vi "Main.vi"() -> ()   [LabVIEW 2013]
uses:
  <vilib>/Utility/error.llb/DialogType.ctl
panel:
  in  "IP":string="192.168.1.4"
  in  "SetRemote":bool
  in  "Сброс ERR":bool
  in  "График":bool
  in  "Voltage 2":u8 caption="мА" max=24 step=1
  in  "SetIB":bool
  in  "Voltage":dbl caption="кВ" min=0.0 max=50.0 step=0.1 format="%.1g"
  in  "SetUB":bool
  out "Режим":bool
  out "Статус":bool
  out "Блок.":bool
  out "Uвых":dbl(graph)
  out "мА":string
  out "Выход":bool
  in  "вкл.":bool
  out "conn src":refnum<k5>
  in  "stop":bool
  out "message":string=" INSTRUCTIONS:\r\rNormal Use:  When using subVIs that incorporate the error in/error out (or error I/O) structure, place this handler where you want to inform the user of an error, typically at the end of the I/O data path, as the last action of the program.  If the error in error? is ERROR, the handler creates a message describing the error and its source.  If the type of dialog = 1 (default), the message is displayed to the user, who can only acknowedge it.  If the type = 2, the user can acknowledge the message or abort execution; aborting a program with active I/O is not recommended.  If the type = 0, no message is displayed; this is used to process the error programmatically, and the error out cluster elements are wired to individual terminals for that reason.  \r\rOther Use:\n\r\nlocal testing.  To test the error code of a subVI or function that does not have the error I/O structure, you can wire its error code and a source string to the local error code and error source inputs.  If error in error? indicates no error and error code is not equal to 0, the local code and source are substituted for the error in values, and error? is set TRUE (ERROR)."
  out "кВ":string
  # "SPELLMAN 50 кВ 24 мА"
  # "Установки"
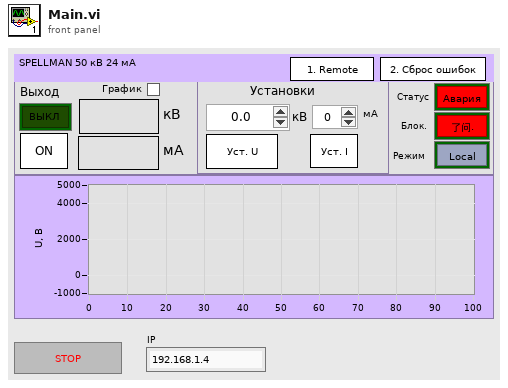
[diagram p1: front panel]
types:
  T1 = typedef "DialogType.ctl" = u16
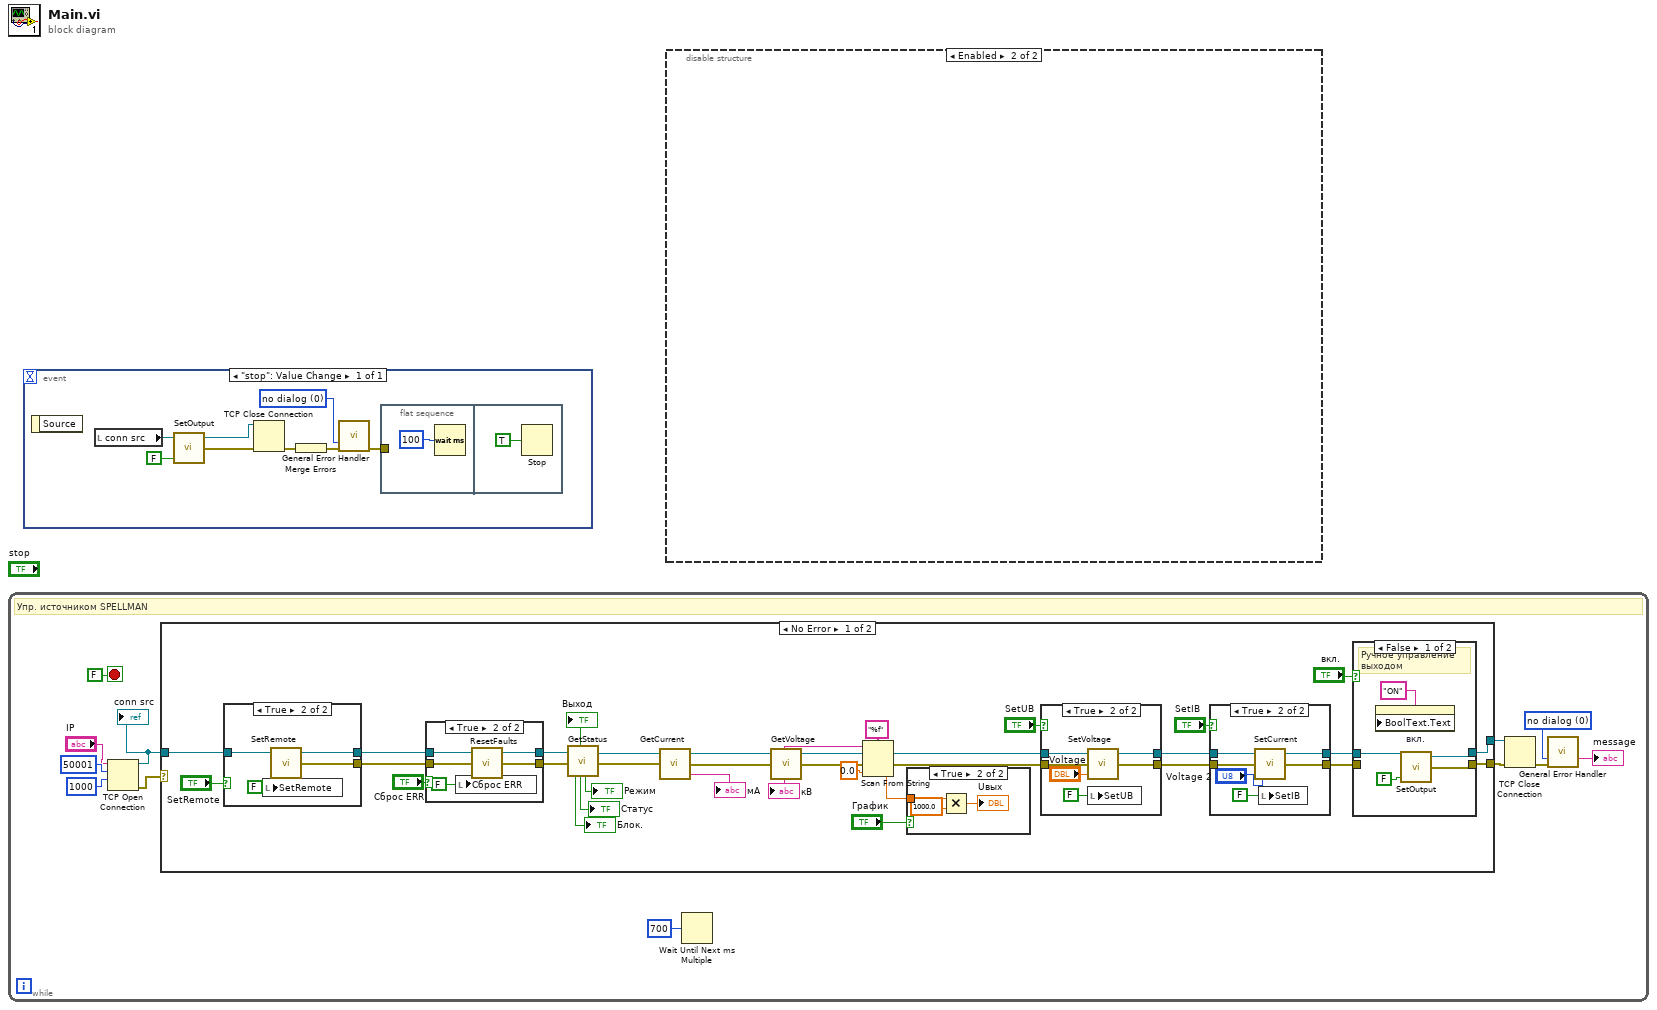
[diagram p0: block diagram]
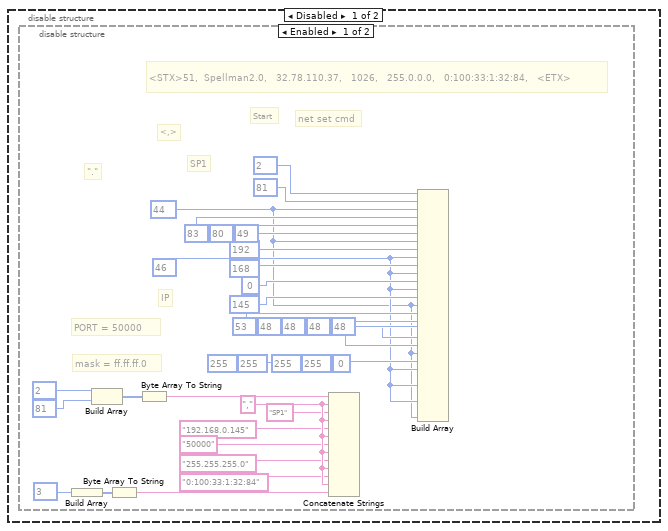
[diagram p2: hidden frame]
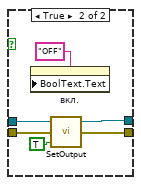
[diagram p9: hidden frame]
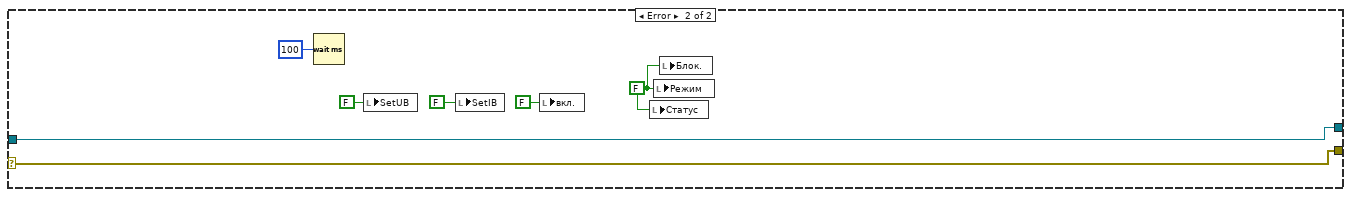
[diagram p10: hidden frame]
diagram:
  n1 = while {
    stop <- FALSE stop-if-true
    w9 = T1 0 items=["no dialog", "OK message", "continue or stop message", "OK message + warnings", "continue/stop + warnings"] ("type of dialog (OK msg:1)")
    # "Упр. источником SPELLMAN"
    n2 = TCP Open Connection(address="IP", remote port or service name=u16 50001 ("Port"), timeout ms (60000)=1000) -> (connection ID=w3:refnum<k5>, error out=w2:errorcluster)  [unwired: 2 in]
    "conn src" <- w3
    n3 = case shown="No Error" w2 {
      selector: w2 -> [_ w92]
      tunnel: w3 -> [w15 w93]
      tunnel: [w45 w93] -> w12
      tunnel: [w44 w92] -> w11
      frame No Error {
        n4 = case shown="True" "SetRemote" {
          tunnel: [w46 w50] -> w16
          tunnel: w15 -> [w46 w49]
          tunnel: [_ w48] -> w14
          frame False {
          }
          frame True {
            n5 = local write "SetRemote"(FALSE ("SetRemote")) -> ()
            n6 = call "SetRemote.vi"("connection ID"=w49) -> ("error out"=w48:errorcluster, "connection ID out"=w50:refnum<k5>)  [unwired: 2 in, 1 out]
          }
        }
        n7 = case shown="True" "Сброс ERR" {
          tunnel: w16 -> [w52 w57]
          tunnel: [w52 w56] -> w17
          tunnel: [w51 w55] -> w18
          tunnel: w14 -> [w51 w53]
          frame False {
          }
          frame True {
            n8 = local write "Сброс ERR"(FALSE ("Сброс ERR")) -> ()
            n9 = call "ResetFaults.vi"("error in"=w53, "connection ID"=w57) -> ("error out"=w55:errorcluster, "connection ID out"=w56:refnum<k5>)  [unwired: 1 in, 1 out]
          }
        }
        n10 = call "GetStatus.vi"("connection ID in"=w17, "error in"=w18) -> ("InterlLoc State"=→"Блок.":bool, "OutState"=→"Выход":bool, "Fault"=→"Статус":bool, "Rem|Loc"=→"Режим":bool, "connection ID out"=w25:refnum<k5>, "error out"=w24:errorcluster)  [unwired: 12 in]
        n11 = call "GetCurrent.vi"("error in"=w24, "connection ID"=w25) -> ("Current"=→"мА":string, "error out"=w42:errorcluster, "connection ID out"=w41:refnum<k5>)  [unwired: 1 out]
        n12 = call "GetVoltage.vi"("error in"=w42, "connection ID"=w41) -> ("Voltage"=w36:string, "error out"=w33:errorcluster, "connection ID out"=w40:refnum<k5>)  [unwired: 1 out]
        "кВ" <- w36
        n13 = Scan From String(format string="%f", input string=w36, error in=w33, default 1=0.0 ("default (0 I32)")) -> (error out=w32:errorcluster, output 1=w34:dbl)  [unwired: 1 in, 2 out]
        n14 = case shown="True" "График" {
          tunnel: w34 -> [_ w58]
          frame False {
          }
          frame True {
            n15 = Multiply(x=w58, y=1000.0) -> (x*y=→"Uвых":dbl)
          }
        }
        n16 = case shown="True" "SetUB" {
          tunnel: w32 -> [w70 w76]
          tunnel: [w70 w75] -> w29
          tunnel: w40 -> [w69 w74]
          tunnel: [w69 w72] -> w30
          frame False {
          }
          frame True {
            n17 = call "SetVoltage.vi"("Voltage"="Voltage", "error in"=w76, "connection ID"=w74) -> ("error out"=w75:errorcluster, "connection ID out"=w72:refnum<k5>)  [unwired: 1 out]
            n18 = local write "SetUB"(FALSE ("SetUB")) -> ()
          }
        }
        n19 = case shown="True" "SetIB" {
          tunnel: w30 -> [w62 w67]
          tunnel: w29 -> [w61 w66]
          tunnel: [w61 w65] -> w28
          tunnel: [w62 w64] -> w27
          frame False {
          }
          frame True {
            n20 = call "SetCurrent.vi"("Current"="Voltage 2", "error in"=w66, "connection ID in"=w67) -> ("error out"=w65:errorcluster, "connection ID out"=w64:refnum<k5>)  [unwired: 1 out]
            n21 = local write "SetIB"(FALSE ("SetUB")) -> ()
          }
        }
        n22 = case shown="False" "вкл." {
          tunnel: [w80 w85] -> w45
          tunnel: [w79 w84] -> w44
          tunnel: w28 -> [_ w83]
          tunnel: w27 -> [w77 w82]
          frame False {
            # "Ручное управление выходом"
            n23 = property on="вкл." class="Bool (strict)"("BoolText.Text"="ON") -> ()  [unwired: 2 in, 2 out]
            n24 = call "SetOutput.vi"("State"=FALSE, "connection ID"=w77) -> ("error out"=w79:errorcluster, "connection ID out"=w80:refnum<k5>)  [unwired: 2 in]
          }
          frame True {
            n25 = property on="вкл." class="Bool (strict)"("BoolText.Text"="OFF") -> ()  [unwired: 2 in, 2 out]
            n26 = call "SetOutput.vi"("State"=TRUE, "error in"=w83, "connection ID"=w82) -> ("error out"=w84:errorcluster, "connection ID out"=w85:refnum<k5>)  [unwired: 1 in]
          }
        }
      }
      frame Error {
        w88 = FALSE ("Режим")
        n27 = Wait (ms)(milliseconds to wait=u32 100) -> ()  [unwired: 1 out]
        n28 = local write "SetUB"(FALSE ("SetUB")) -> ()
        n29 = local write "SetIB"(FALSE ("SetUB")) -> ()
        n30 = local write "вкл."(FALSE ("вкл.")) -> ()
        n31 = local write "Статус"(w88) -> ()
        n32 = local write "Режим"(w88) -> ()
        n33 = local write "Блок."(w88) -> ()
      }
    }
    n34 = Wait Until Next ms Multiple(millisecond multiple=u32 700 ("milliseconds to wait")) -> ()  [unwired: 1 out]
    n35 = TCP Close Connection(connection ID=w12, error in (no error)=w11) -> (error out=w10:errorcluster)  [unwired: 2 out]
    n36 = call <vilib>:"General Error Handler.vi"("type of dialog (OK msg:1)"=w9, "error in (no error)"=w10) -> ("message"=→"message":string)  [unwired: 9 in, 4 out]
  }
  n37 = event shown="[0] \"stop\": Value Change" {
    selector: _ -> [_]
    dyn-events: _ -> [_]
    timeout: _ -> [_]
    event "stop": Value Change {
      w100 = T1 0 items=["no dialog", "OK message", "continue or stop message", "OK message + warnings", "continue/stop + warnings"] ("type of dialog (OK msg:1)")
      n38 = event-data() -> ()  [unwired: 1 in, 1 out]
      n39 = local read "conn src"() -> (w98:refnum<k5>)
      n40 = call "SetOutput.vi"("State"=FALSE, "connection ID"=w98) -> ("error out"=w96:errorcluster, "connection ID out"=w97:refnum<k5>)  [unwired: 1 in, 1 out]
      n41 = TCP Close Connection(connection ID=w97, error in (no error)=w96) -> (error out=w102:errorcluster)  [unwired: 1 in, 1 out]
      n42 = Merge Errors(w102) -> (w101:errorcluster)
      n43 = call <vilib>:"General Error Handler.vi"("type of dialog (OK msg:1)"=w100, "error in (no error)"=w101) -> ("error out"=w99:errorcluster)  [unwired: 9 in, 4 out]
      n44 = flat-sequence {
        tunnel: w99 -> [_]
        frame #0 {
          n45 = Wait (ms)(milliseconds to wait=u32 100) -> ()  [unwired: 1 out]
        }
        frame #1 {
          n46 = Stop(stop? (T)=TRUE) -> ()
        }
      }
    }
  }
  n47 = disable-structure shown="Enabled" {
    frame Disabled {
      n48 = disable-structure shown="Enabled" {
        frame Enabled {
          w114 = "," ("string")
          (unwired) u8 0 ("y")
          (unwired) u8 255 ("y")
          (unwired) u8 255 ("y")
          (unwired) u8 255 ("y")
          w119 = u8 46 ("y")
          w118 = u8 44 ("y")
          # "mask = ff.ff.ff.0"
          # "PORT = 50000"
          # "IP"
          # "\".\""
          # "net set cmd"
          # "Start"
          # "<,>"
          # "SP1"
          # "<STX>51,  Spellman2.0,   32.78.110.37,   1026,   255.0.0.0,   0:100:33:1:32:84,   <ETX>"
          n49 = Build Array(u8 3 ("y")) -> (w116:u8[])
          n50 = Build Array(u8 2 ("y"), u8 81 ("y")) -> (w105:u8[])
          n51 = Byte Array To String(unsigned byte array=w116) -> (string=w117:string)
          n52 = Byte Array To String(unsigned byte array=w105) -> (string=w108:string)
          n53 = Concatenate Strings(w108, w114, "SP1" ("string"), w114, "192.168.0.145", w114, "50000", w114, "255.255.255.0", w114, "0:100:33:1:32:84", w114, w117) -> ()  [unwired: 1 out]
          n54 = Build Array(u8 2 ("y"), u8 81 ("y"), w118, u8 83 ("y"), u8 80 ("y"), u8 49 ("y"), w118, u8 192 ("y"), w119, u8 168 ("y"), w119, u8 0 ("y"), w119, u8 145 ("y"), w118, u8 53 ("y"), u8 48 ("y"), u8 48 ("y"), u8 48 ("y"), u8 48 ("y"), w118, u8 255 ("y"), w119, w119, w119, w118) -> ()  [unwired: 3 in, 1 out]
        }
        frame Disabled {
        }
      }
    }
    frame Enabled {
    }
  }
